vi "Test Assert True.vi"(8 "error in (no error)":errorcluster) -> (0 "error out":errorcluster)   [LabVIEW 2009]
uses:
  classes/Assert/Assert.lvclass
  classes/Test/Test.lvclass
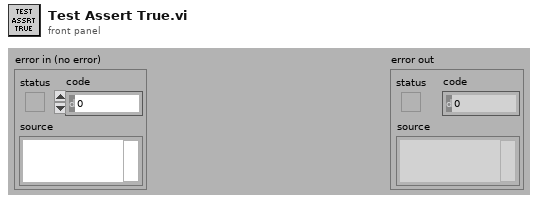
[diagram p1: front panel]
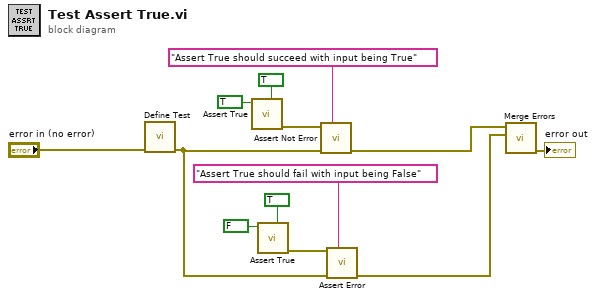
[diagram p0: block diagram]
diagram:
  n1 = call "Define Test.vi"("error in (no error)"="error in (no error)") -> ("error out"=w1:errorcluster)  [unwired: 10 in]
  n2 = call "Assert True.vi"("Assert Only? (F)"=TRUE, "True?"=TRUE) -> ("error out"=w12:errorcluster)  [unwired: 9 in]
  n3 = call "Assert True.vi"("Assert Only? (F)"=TRUE, "True?"=FALSE) -> ("error out"=w9:errorcluster)  [unwired: 9 in]
  n4 = call "Assert Not Error.vi"("Label"="Assert True should succeed with input being True", "error in (no error)"=w1, "Not Error?"=w12) -> ("error out"=w3:errorcluster)  [unwired: 8 in]
  n5 = call "Assert Error.vi"("Label"="Assert True should fail with input being False", "error in (no error)"=w1, "Error?"=w9) -> ("error out"=w4:errorcluster)  [unwired: 8 in]
  n6 = call <vilib>:"Merge Errors.vi"("error in 2 (no error)"=w4, "error in 1 (no error)"=w3) -> ("error out"=→"error out":errorcluster)  [unwired: 5 in]
